vi "WriteHeadersCsv.vi"(0 "session in":refnum<k35>, 11 "error in":errorcluster) -> (4 "session out":refnum<k35>, 15 "error out":errorcluster)   [LabVIEW 2023]
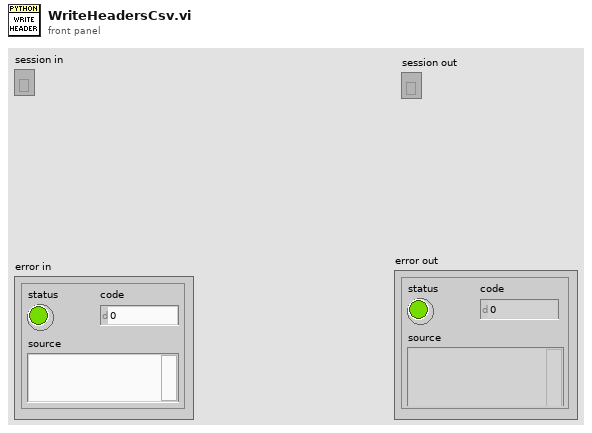
[diagram p1: front panel]
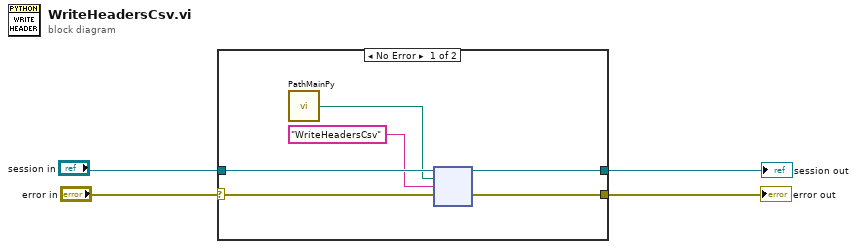
[diagram p0: block diagram]
diagram:
  n1 = case shown="No Error" "error in" {
    selector: "error in" -> [w10 w12]
    tunnel: [w8 w12] -> w4
    tunnel: "session in" -> [w9 w11]
    tunnel: [w7 w11] -> w1
    frame No Error {
      n2 = call "PathMainPy.vi"() -> ("path"=w5:path)  [unwired: 15 in]
      n3 = node(w9, w5, "WriteHeadersCsv" ("function name"), w10) -> (w7:refnum<k35>, w8:errorcluster)  [unwired: 2 in, 2 out]
    }
    frame Error {
    }
  }
  "error out" <- w4
  "session out" <- w1
